vi "READ FROM SINGLE ROW.vi"(8 "error in (no error)":errorcluster, 11 "id Manual":i32) -> (0 "error out":errorcluster, 1 "Analog - Digital":bool, 2 "ANALOGICO":T2={"ANALOGICO CANALES"=[], "Numero de muestras"=1000, "Frecuencia de muestreo"=1000}, 3 "DIGITAL":T1={"Puertos Digital"=[], "Lineas Digital"=[], "Frecuencia Muestreo"=1000, "Puerto/Linea"=FALSE}, 4 "DAQ Device Name":tag, 5 "Total Acquisition Time":i32)   [LabVIEW 2020, in "Settings.lvlib"]
uses:
  Settings.lvlib
  Acquisition/cluster analogico.ctl
  Acquisition/cluster digital.ctl
  <vilib>/drjdpowell/SQLite Library/SQL Connection/Open (path).vi
  <vilib>/drjdpowell/SQLite Library/SQL Connection/Open (string).vi
  <vilib>/AdvancedString/Path To Command Line String.vi
  <vilib>/drjdpowell/SQLite Library/SQL Connection/Execute SQL (1D String).vi
  <vilib>/drjdpowell/SQLite Library/SQL Connection/Connection.lvclass
  <vilib>/drjdpowell/SQLite Library/SQLite.lvlib
  Acquisition/CONTROLS.lvlib
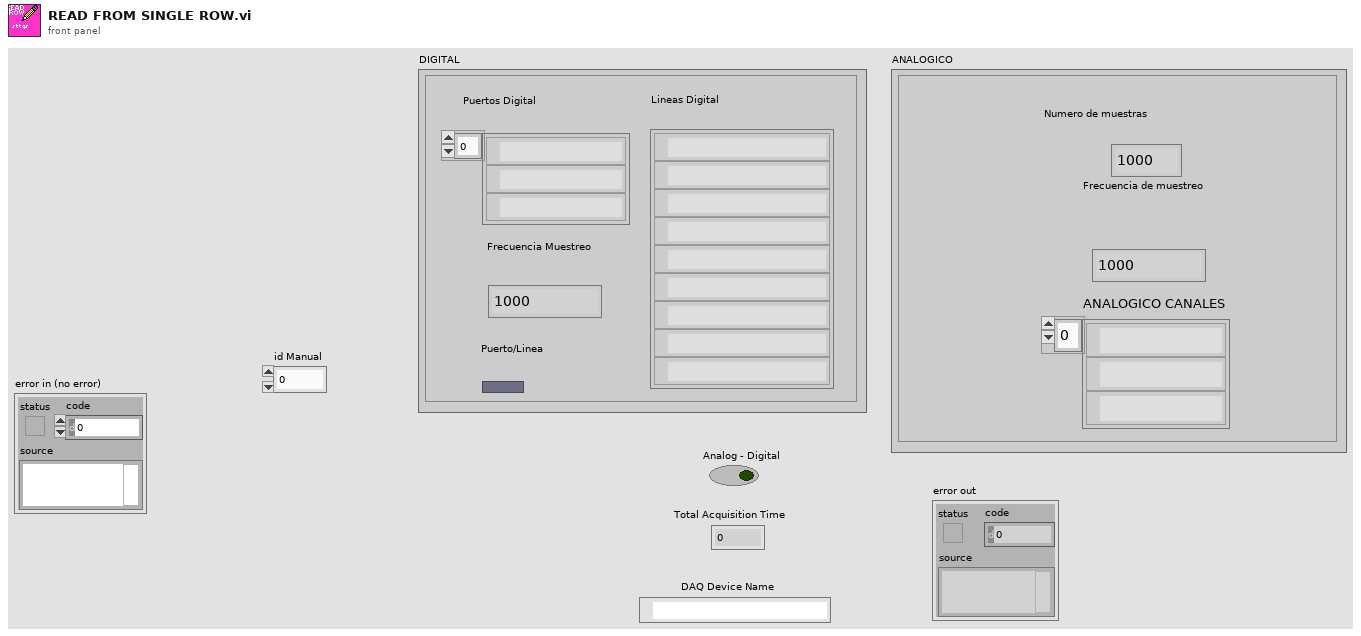
[diagram p1: front panel]
types:
  T1 = typedef "Acquisition.lvlib/CONTROLS.lvlib/cluster digital.ctl" = cluster{"Puertos Digital":tag[], "Lineas Digital":tag[], "Frecuencia Muestreo":u32, "Puerto/Linea":bool}
  T2 = typedef "Acquisition.lvlib/CONTROLS.lvlib/cluster analogico.ctl" = cluster{"ANALOGICO CANALES":tag[], "Numero de muestras":u32, "Frecuencia de muestreo":u32}
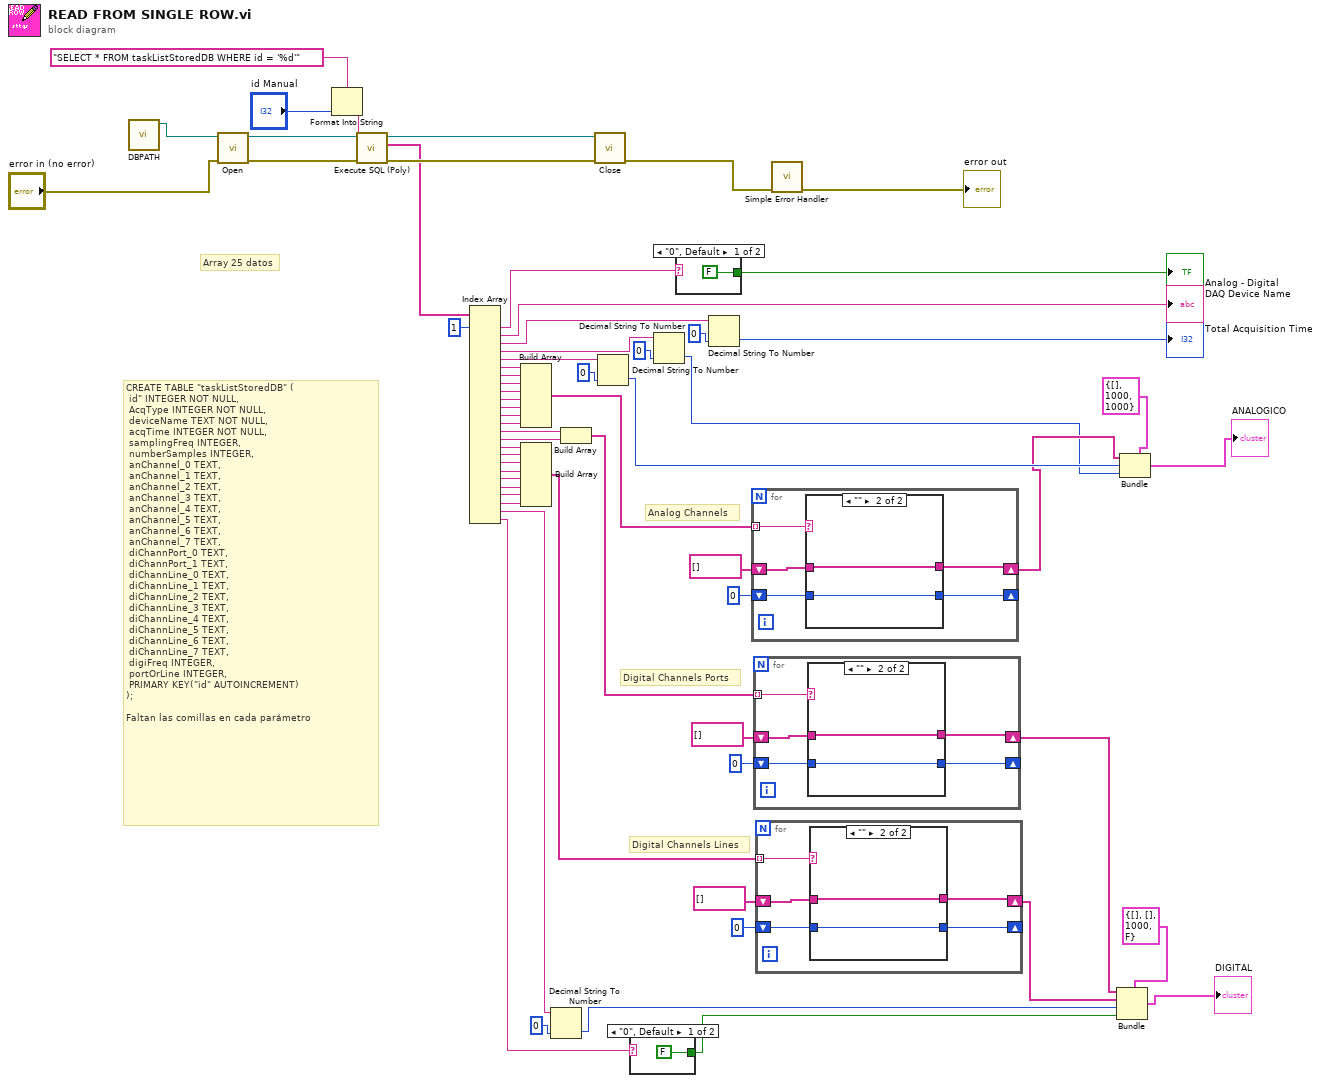
[diagram p0: block diagram]
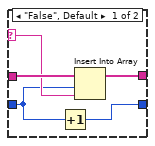
[diagram p2: hidden frame]
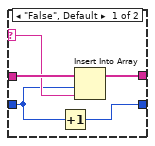
[diagram p3: hidden frame]
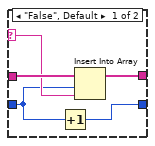
[diagram p4: hidden frame]
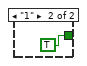
[diagram p5: hidden frame]
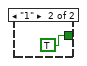
[diagram p6: hidden frame]
diagram:
  # "Digital Channels Lines"
  # "Digital Channels Ports"
  # "Analog Channels"
  # "CREATE TABLE \"taskListStoredDB\" (\n\tid\"\tINTEGER NOT NULL,\n\tAcqType\tINTEGER NOT NULL,\n\tdeviceName\tTEXT NOT NULL,\n\tacqTime\tINTEGER NOT NULL,\n\tsamplingFreq\tINTEGER,\n\tnumberSamples\tINTEGER,\n\tanChannel_0\tTEXT,\n\tanChannel_1\tTEXT,\n\tanChannel_2\tTEXT,\n\tanChannel_3\tTEXT,\n\tanChannel_4 TEXT,\n\tanChannel_5\tTEXT,\n\tanChannel_6\tTEXT,\n\tanChannel_7\tTEXT,\n\tdiChannPort_0\tTEXT,\n\tdiChannPort_1\tTEXT,\n\tdiChannLine_0\tTEXT,\n\tdiChannLine_1\tTEXT,\n\tdiChannLine_2\tTEXT,\n\tdiChannLine_3\tTEXT,\n\tdiChannLine_4\tTEXT,\n\tdiChannLine_5\tTEXT,\n\tdiChannLine_6\tTEXT,\n\tdiChannLine_7\tTEXT,\n\tdigiFreq\tINTEGER,\n\tportOrLine INTEGER,\n\tPRIMARY KEY(\"id\" AUTOINCREMENT)\n);\n\nFaltan las comillas en cada parámetro"
  # "Array 25 datos"
  n1 = call "DBPATH.vi"() -> ("appended path"=w8:path)  [unwired: 11 in]
  n2 = call-poly <vilib>:"Open.vi"("error in (no error)"="error in (no error)", "db file"=w8) -> ("error out"=w64:errorcluster, "SQLite Connection"=w61:refnum<class "Connection.lvclass">)  [unwired: 8 in]
  n3 = Format Into String(format string="SELECT * FROM taskListStoredDB WHERE id = '%d'" ("SQL"), "id Manual") -> (resulting string=w57:string)  [unwired: 2 in, 1 out]
  n4 = call-poly <vilib>:"Execute SQL (Poly).vi"("error in (no error)"=w64, "SQL"=w57, "SQLite Connection in"=w61) -> ("error out"=w62:errorcluster, "Result Set"=w54:string[], "SQLite Connection"=w60:refnum<class "Connection.lvclass">)  [unwired: 5 in, 1 out]
  n5 = Index Array(array=w54, index #1=1 ("index")) -> (element #1=w53:string, element #2=→"DAQ Device Name":string, element #3=w50:string, element #4=w45:string, element #5=w44:string, element #6=w42:string, element #7=w41:string, element #8=w40:string, element #9=w39:string, element #10=w38:string, element #11=w37:string, element #12=w36:string, element #13=w35:string, element #14=w34:string, element #15=w33:string, element #16=w32:string, element #17=w31:string, element #18=w30:string, element #19=w29:string, element #20=w28:string, element #21=w27:string, element #22=w26:string, element #23=w25:string, element #24=w23:string, element #25=w21:string)  [unwired: 24 in]
  n6 = Build Array(w42, w41, w40, w39, w38, w37, w36, w35) -> (w17:string[])
  n7 = Build Array(w32, w31, w30, w29, w28, w27, w26, w25) -> (w10:string[])
  n8 = Decimal String To Number(string=w23, default (0L)=0 ("default (0 I32)")) -> (number=w22:i32)  [unwired: 1 in, 1 out]
  n9 = Build Array(w34, w33) -> (w14:string[])
  n10 = call-dynamic "Close.vi"("error in (no error)"=w62, "SQLite Connection in"=w60) -> ("error out"=w58:errorcluster)  [unwired: 9 in]
  n11 = Decimal String To Number(string=w44, default (0L)=0 ("default (0 I32)")) -> (number=w43:i32)  [unwired: 1 in, 1 out]
  n12 = case shown="\"0\", Default" w21 {
    tunnel: [FALSE TRUE] -> w20
    frame "0", Default {
    }
    frame "1" {
    }
  }
  n13 = Decimal String To Number(string=w45, default (0L)=0 ("default (0 I32)")) -> (number=w3:i32)  [unwired: 1 in, 1 out]
  n14 = case shown="\"0\", Default" w53 {
    tunnel: [FALSE TRUE] -> w52
    frame "0", Default {
    }
    frame "1" {
    }
  }
  "Analog - Digital" <- w52
  n15 = Decimal String To Number(string=w50, default (0L)=0 ("default (0 I32)")) -> (number=→"Total Acquisition Time":i32)  [unwired: 1 in, 1 out]
  n16 = for {
    tunnel: w17 -> [w73] mode=indexing
    shift-right: [w71] -> w4
    shift-left: string[] [] -> [w72]
    shift-right: [w69] -> _
    shift-left: 0 -> [w70]
    n17 = case shown="\"\"" w73 {
      selector: w73 -> [w77 _]
      tunnel: w72 -> [w78 w79]
      tunnel: [w76 w79] -> w71
      tunnel: w70 -> [w75 w80]
      tunnel: [w74 w80] -> w69
      frame "False", Default {
        n18 = Increment(x=w75) -> (x+1=w74:i32)
        n19 = Insert Into Array(array=w78, index=w75, new element=w77) -> (w76:string[])
      }
      frame "" {
      }
    }
  }
  n20 = for {
    tunnel: w14 -> [w85] mode=indexing
    shift-right: [w83] -> w13
    shift-left: string[] [] -> [w84]
    shift-right: [w81] -> _
    shift-left: 0 -> [w82]
    n21 = case shown="\"\"" w85 {
      selector: w85 -> [w89 _]
      tunnel: w84 -> [w90 w91]
      tunnel: [w88 w91] -> w83
      tunnel: w82 -> [w87 w92]
      tunnel: [w86 w92] -> w81
      frame "False", Default {
        n22 = Increment(x=w87) -> (x+1=w86:i32)
        n23 = Insert Into Array(array=w90, index=w87, new element=w89) -> (w88:string[])
      }
      frame "" {
      }
    }
  }
  n24 = for {
    tunnel: w10 -> [w97] mode=indexing
    shift-right: [w95] -> w9
    shift-left: string[] [] -> [w96]
    shift-right: [w93] -> _
    shift-left: 0 -> [w94]
    n25 = case shown="\"\"" w97 {
      selector: w97 -> [w101 _]
      tunnel: w96 -> [w102 w103]
      tunnel: [w100 w103] -> w95
      tunnel: w94 -> [w99 w104]
      tunnel: [w98 w104] -> w93
      frame "False", Default {
        n26 = Increment(x=w99) -> (x+1=w98:i32)
        n27 = Insert Into Array(array=w102, index=w99, new element=w101) -> (w100:string[])
      }
      frame "" {
      }
    }
  }
  n28 = call <vilib>:"Simple Error Handler.vi"("error in (no error)"=w58) -> ("error out"=→"error out":errorcluster)  [unwired: 4 in, 4 out]
  n29 = Bundle(cluster=T1 {"Puertos Digital"=[], "Lineas Digital"=[], "Frecuencia Muestreo"=1000, "Puerto/Linea"=FALSE} ("DIGITAL"), "Puertos Digital"=w13, "Lineas Digital"=w9, "Frecuencia Muestreo"=w22, "Puerto/Linea"=w20) -> (→"DIGITAL":T1)
  n30 = Bundle(cluster=T2 {"ANALOGICO CANALES"=[], "Numero de muestras"=1000, "Frecuencia de muestreo"=1000} ("ANALOGICO"), "ANALOGICO CANALES"=w4, "Numero de muestras"=w43, "Frecuencia de muestreo"=w3) -> (→"ANALOGICO":T2)
